vi "Dynamic Resizing.vi"() -> ()   [LabVIEW 2012]
uses:
  vi.lib/Front Panel Layout/Scaling Settings.ctl
  vi.lib/Front Panel Layout/Scaling Type.ctl
  vi.lib/Front Panel Layout/VI Panel Layout/VI Panel Layout.lvclass
  vi.lib/Front Panel Layout/NI_SE_Front Panel Layout.lvlib
panel:
  in  "Listbox":i32(listbox)
  in  "String":string
  in  "cancel":bool
  in  "ok":bool
  in  "Scale Text":bool
  in  "Data":dbl
  in  "Param2":dbl
  in  "Param1":dbl
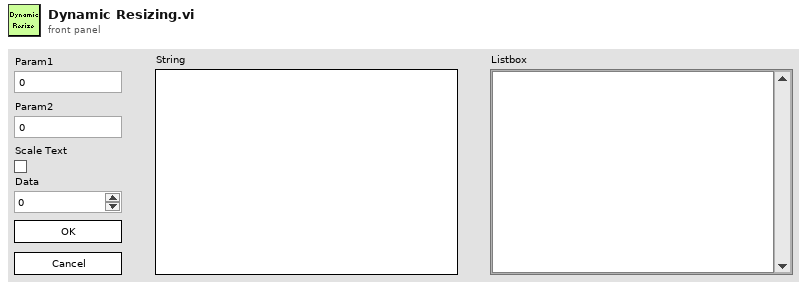
[diagram p1: front panel]
types:
  T1 = typedef "NI_SE_Front Panel Layout.lvlib/Scaling Type.ctl" = enum16{"None", "Scale panel to fit layout", "Scale layout to fit panel"}
  T2 = typedef "NI_SE_Front Panel Layout.lvlib/Scaling Settings.ctl" = cluster{"scaling type":T1, "scale text":bool}
  T3 = typedef "LVRectTypeDef.ctl" = cluster{"Left":i16, "Top":i16, "Right":i16, "Bottom":i16}
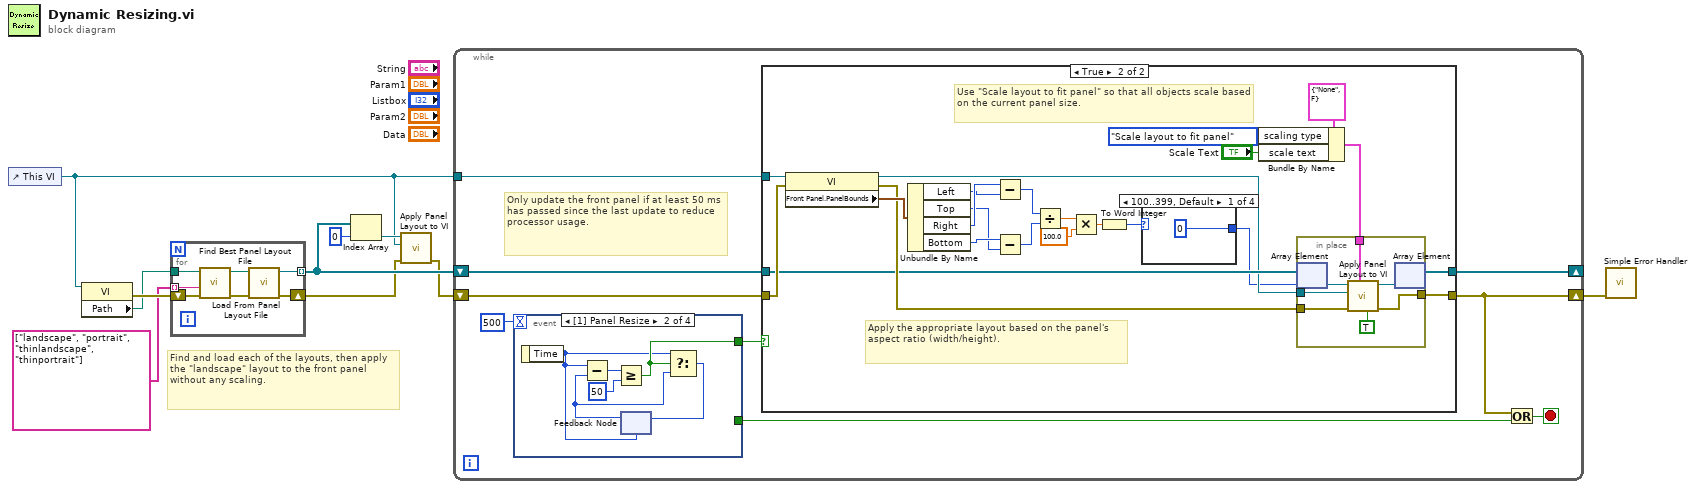
[diagram p0: block diagram]
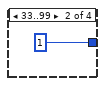
[diagram p3: hidden frame]
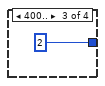
[diagram p4: hidden frame]
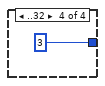
[diagram p5: hidden frame]
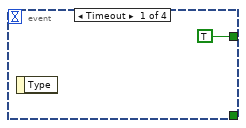
[diagram p6: hidden frame]
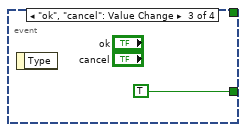
[diagram p7: hidden frame]
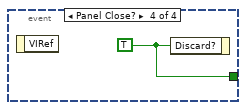
[diagram p8: hidden frame]
diagram:
  # "Find and load each of the layouts, then apply the \"landscape\" layout to the front panel without any scaling."
  n1 = control-ref of="This VI"() -> (w3:refnum<vi>)
  n2 = property class="VI"(reference=w3) -> (error out=w10:errorcluster, "Path"=w9:path)  [unwired: 1 in, 1 out]
  n3 = for {
    tunnel: w9 -> [w16]
    tunnel: string[] ["landscape", "portrait", "thinlandscape", "thinportrait"] -> [w13] mode=indexing
    shift-right: [w12] -> w5
    shift-left: w10 -> [w17]
    tunnel: [w11] -> w7 mode=indexing
    n4 = call "Find Best Panel Layout File.vi"("error in"=w17, "keyword to match (\"\")"=w13, "VI path"=w16) -> ("error out"=w14:errorcluster, "panel layout file"=w15:path)  [unwired: 6 in, 1 out]
    n5 = call "Load From Panel Layout File.vi"("error in"=w14, "panel layout file"=w15) -> ("error out"=w12:errorcluster, "panel layout out"=w11:refnum<class "VI Panel Layout.lvclass">)  [unwired: 8 in]
  }
  n6 = Index Array(array=w7, index=0) -> (element=w6:refnum<class "VI Panel Layout.lvclass">)
  n7 = call "Apply Panel Layout to VI.vi"("error in"=w5, "VI refnum"=w3, "panel layout in"=w6) -> ("error out"=w4:errorcluster)  [unwired: 7 in, 1 out]
  n8 = while {
    shift-right: [w18] -> w1
    shift-left: w4 -> [w24]
    tunnel: w3 -> [w20]
    shift-right: [w19] -> _
    shift-left: w7 -> [w23]
    stop <- w22 stop-if-true
    # "Only update the front panel if at least 50 ms has passed since the last update to reduce processor usage."
    n9 = event shown="[1] Panel Resize" {
      selector: _ -> [_ _ _ _]
      dyn-events: _ -> [_ _ _ _]
      timeout: 500 -> [_ _ _ _]
      tunnel: [_ _ TRUE w71] -> w21
      tunnel: [TRUE w67 _ _] -> w25
      event Timeout {
        n10 = event-data() -> ()  [unwired: 1 in, 1 out]
      }
      event Panel Resize {
        n11 = event-data() -> ("Time"=w64:u32)  [unwired: 1 in]
        n12 = feedback #1(w64) -> (w66:u32)
        n13 = Subtract(x=w64, y=w66) -> (x-y=w69:u32)
        n14 = Greater Or Equal?(x=w69, y=u32 50) -> (x >= y?=w67:bool)
        n15 = Select(t=w64, s=w67, f=w66) -> (s? t:f=w65:u32)
        n16 = feedback-in #1(w65) -> ()
      }
      event "ok", "cancel": Value Change {
        n17 = event-data() -> ()  [unwired: 1 in, 1 out]
      }
      event Panel Close? {
        w71 = TRUE ("Discard?")
        n18 = event-data() -> ()  [unwired: 1 in, 1 out]
        n19 = event-data("Discard?"=w71) -> ()  [unwired: 1 in, 1 out]
      }
    }
    n20 = case shown="True" w25 {
      tunnel: w24 -> [w28 w50]
      tunnel: [w28 w43] -> w18
      tunnel: w23 -> [w27 w38]
      tunnel: w20 -> [_ w51]
      tunnel: [w27 w37] -> w19
      frame False {
      }
      frame True {
        # "Use \"Scale layout to fit panel\" so that all objects scale based on the current panel size."
        # "Apply the appropriate layout based on the panel's aspect ratio (width/height)."
        n21 = property class="VI"(reference=w51, error in=w50) -> (reference out=w36:refnum<vi>, error out=w44:errorcluster, "Front Panel.PanelBounds"=w49:T3)
        n22 = Unbundle By Name(w49) -> ("Left"=w47:i16, "Top"=w45:i16, "Right"=w48:i16, "Bottom"=w46:i16)
        n23 = Subtract(x=w48, y=w47) -> (x-y=w35:i16)
        n24 = Subtract(x=w46, y=w45) -> (x-y=w34:i16)
        n25 = Divide(x=w35, y=w34) -> (x/y=w33:dbl)
        n26 = Multiply(x=w33, y=100.0) -> (x*y=w31:dbl)
        n27 = To Word Integer(number=w31) -> (16bit integer=w30:i16)
        n28 = case shown="100..399, Default" w30 {
          tunnel: [0 ("index") 1 ("index") 2 ("index") 3 ("index")] -> w29
          frame 100..399, Default {
          }
          frame 33..99 {
          }
          frame 400.. {
          }
          frame ..32 {
          }
        }
        n29 = Bundle By Name(cluster=T2 {"scaling type"=enum."None", "scale text"=FALSE} ("scaling settings"), "scaling type"=Scaling_Type."Scale layout to fit panel", "scale text"="Scale Text") -> (w41:T2)
        n30 = in-place {
          in-place-border: w36 -> [w62]
          in-place-border: w44 -> [w61]
          in-place-border: [w60] -> w43
          in-place-border: w41 -> [w59]
          n31 = in-place-array #2(w38, w29) -> (w58:refnum<class "VI Panel Layout.lvclass">)
          n32 = call "Apply Panel Layout to VI.vi"("defer panel updates (F)"=TRUE ("defer front panel updates (F)"), "scaling settings"=w59, "error in"=w61, "VI refnum"=w62, "panel layout in"=w58) -> ("error out"=w60:errorcluster, "panel layout out"=w57:refnum<class "VI Panel Layout.lvclass">)  [unwired: 5 in]
          n33 = in-place-array #2(w57) -> (w37:refnum<class "VI Panel Layout.lvclass">[])  [unwired: 1 out]
        }
      }
    }
    n34 = Or(x=w18, y=w21) -> (x .or. y?=w22:bool)
  }
  n35 = call <vilib>:"Simple Error Handler.vi"("error in (no error)"=w1) -> ()  [unwired: 4 in, 5 out]
